vi "CRYReport Pic Get Current Position.vi"(10 "CurrentInputPosition":variant) -> (0 "InputPos_Out":i32[](array[numeric]), 2 "sData_Out":string)   [LabVIEW 2013]
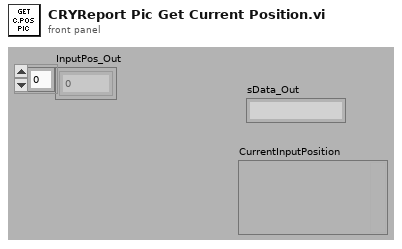
[diagram p1: front panel]
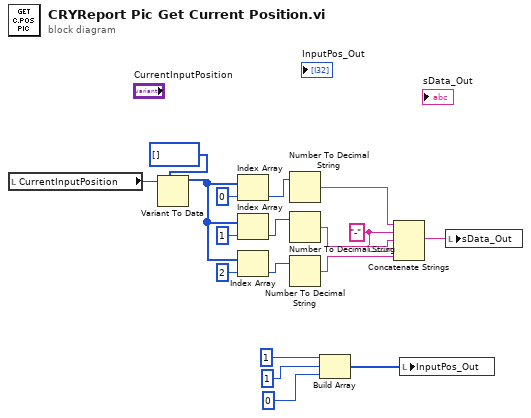
[diagram p0: block diagram]
diagram:
  w9 = "-" ("string")
  n1 = local read "CurrentInputPosition"() -> (w6:variant)
  n2 = Variant To Data(type=i32[] [], Variant=w6) -> (data=w5:i32[])  [unwired: 1 in, 1 out]
  n3 = Index Array(array=w5, index=0) -> (element=w12:i32)
  n4 = Index Array(array=w5, index=1) -> (element=w14:i32)
  n5 = Index Array(array=w5, index=2) -> (element=w13:i32)
  n6 = Number To Decimal String(number=w12) -> (decimal integer string=w11:string)  [unwired: 1 in]
  n7 = Number To Decimal String(number=w14) -> (decimal integer string=w10:string)  [unwired: 1 in]
  n8 = Number To Decimal String(number=w13) -> (decimal integer string=w8:string)  [unwired: 1 in]
  n9 = Build Array(1, 1, 0) -> (w1:i32[])
  n10 = Concatenate Strings(w11, w9, w10, w9, w8) -> (w7:string)
  n11 = local write "InputPos_Out"(w1) -> ()
  n12 = local write "sData_Out"(w7) -> ()
